vi "DriveJoystickButtonMapping.vi"(10 "Joystick Values":dbl[](array[numeric]), 11 "drive joystick buttons":bool[](array[boolean])) -> (3 "output cluster":T1, 4 "drive joystick buttons indicator":bool[](array[boolean]))   [LabVIEW 2019]
uses:
  Controls/DriveJoystickData.ctl
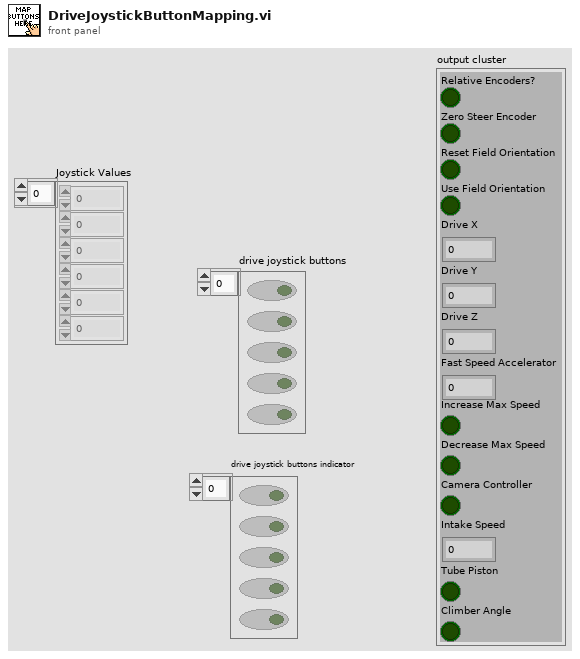
[diagram p1: front panel]
types:
  T1 = typedef "DriveJoystickData.ctl" = cluster{"Relative Encoders?":bool, "Zero Steer Encoder":bool, "Reset Field Orientation":bool, "Use Field Orientation":bool, "Drive X":dbl, "Drive Y":dbl, "Drive Z":dbl, "Fast Speed Accelerator":dbl, "Increase Max Speed":bool, "Decrease Max Speed":bool, "Camera Controller":bool, "Intake Speed":dbl, "Tube Piston":bool, "Climber Angle":bool}
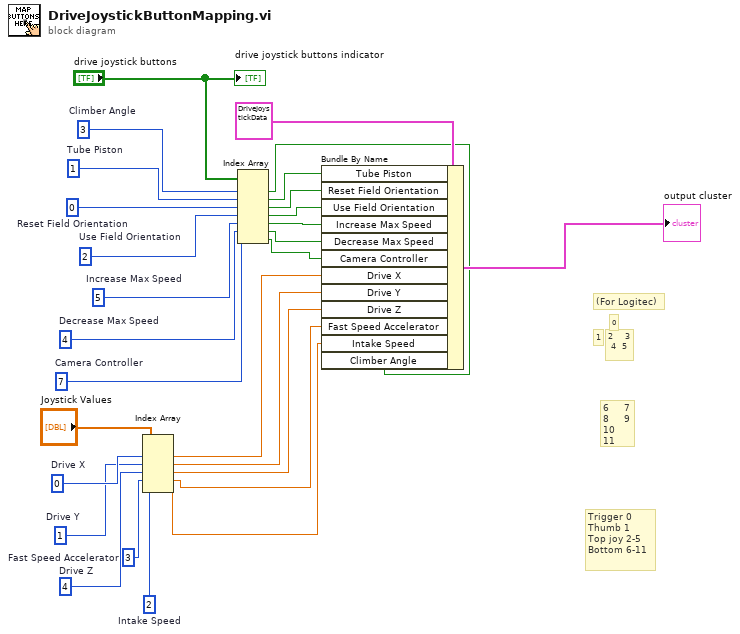
[diagram p0: block diagram]
diagram:
  w2 = 3  # Climber Angle
  w3 = 1  # Tube Piston
  w6 = 2  # Intake Speed
  w9 = 7  # Camera Controller
  w7 = 3  # Fast Speed Accelerator
  w12 = 4  # Drive Z
  w13 = 1  # Drive Y
  w14 = 0  # Drive X
  w15 = 4  # Decrease Max Speed
  w21 = 5  # Increase Max Speed
  w27 = 2  # Use Field Orientation
  w28 = 0  # Reset Field Orientation
  # "(For Logitec)"
  # "6     7\n8     9\n10  11"
  # "2    3\n 4  5"
  # "1"
  # "0"
  # "Trigger 0\nThumb 1\nTop joy 2-5\nBottom 6-11"
  n1 = Index Array(array="Joystick Values", index #1=w14, index #2=w13, index #3=w12, index #4=w7, index #5=w6) -> (element #1=w11:dbl, element #2=w18:dbl, element #3=w17:dbl, element #4=w8:dbl, element #5=w5:dbl)
  n2 = Index Array(array="drive joystick buttons", index #1=w2, index #2=w3, index #3=w28, index #4=w27, index #5=w21, index #6=w15, index #7=w9) -> (element #1=w1:bool, element #2=w4:bool, element #3=w25:bool, element #4=w24:bool, element #5=w20:bool, element #6=w16:bool, element #7=w10:bool)
  n3 = Bundle By Name(cluster=T1 {"Relative Encoders?"=FALSE, "Zero Steer Encoder"=FALSE, "Reset Field Orientation"=FALSE, "Use Field Orientation"=FALSE, "Drive X"=0.0, "Drive Y"=0.0, "Drive Z"=0.0, "Fast Speed Accelerator"=0.0, "Increase Max Speed"=FALSE, "Decrease Max Speed"=FALSE, "Camera Controller"=FALSE, "Intake Speed"=0.0, "Tube Piston"=FALSE, "Climber Angle"=FALSE} ("DriveJoystickButtonMapping"), "Tube Piston"=w4, "Reset Field Orientation"=w25, "Use Field Orientation"=w24, "Increase Max Speed"=w20, "Decrease Max Speed"=w16, "Camera Controller"=w10, "Drive X"=w11, "Drive Y"=w18, "Drive Z"=w17, "Fast Speed Accelerator"=w8, "Intake Speed"=w5, "Climber Angle"=w1) -> (→"output cluster":T1)
  "drive joystick buttons indicator" <- "drive joystick buttons"
